vi "PH_Beamline.color ns-FE BL.vi"(0 "i ref in":refnum<vi>, 5 "error in (no error)":errorcluster) -> (14 "i ref out":refnum<vi>, 16 "Color State Exit ns-FE":i32, 19 "error out":errorcluster)   [LabVIEW 2014, in "PH_Beamline.lvlib"]
doc: "This VI colors the ns-Frontend beamline elements."
uses:
  PH_Beamline.lvlib
  PH_Basics/PH_SystemInformation/PH_SystemInformationEnabling State.ctl
  PH_Basics/PH_StatusHandler/PH_StatusHandler.Status.ctl
  PH_Basics/PH_Common/PH_Common.lvlib
  PH_Basics/PH_SystemInformation/PH_SystemInformation.lvlib
  PH_BL-Master/PH_BL-Master.lvlib
  PH_Basics/PH_StatusHandler/PH_StatusHandler.lvlib
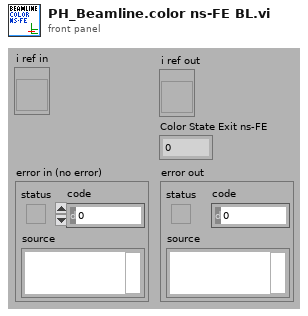
[diagram p1: front panel]
types:
  T1 = enum16{"Laser", "PreAmp", "MainAmp", "Exp 1", "Exp 2", "Exp 3", "Exp 4"}
  T2 = typedef "PH_StatusHandler.lvlib/PH_StatusHandler.Status.ctl" = i16
  T3 = typedef "PH_SystemInformation.lvlib/PH_SystemInformationEnabling State.ctl" = i32
  T4 = typedef "PH_Beamline.lvlib/PH_Beamline.i attribute.ctl" = cluster{"GUI Refs":cluster{"PA ok":refnum<vi>, "MA ok":refnum<vi>, "fs FE ok":refnum<vi>, "ns FE ok":refnum<vi>, "PA ED ok":refnum<vi>, "MAS ok":refnum<vi>, "Booster ok":refnum<vi>, "Mirrortower ok":refnum<vi>, "In.-Box ok":refnum<vi>, "Compressor ok":refnum<vi>, "Experiment LB ok":refnum<vi>, "Experiment LL ok":refnum<vi>, "PHELIX_Beckhoff_Watchdog":refnum<vi>, "Shutters closed":refnum<vi>, "uOPA ok":refnum<vi>, "Vacuum no shotcond Comp LB":refnum<vi>}, "Refs BL MA":refnum<vi>[], "Refs BL MA-IB":refnum<vi>[], "Refs BL fs":refnum<vi>[], "Refs BL PA ED":refnum<vi>[], "Refs BL MAS":refnum<vi>[], "Refs BL Boo":refnum<vi>[], "Refs BL ns":refnum<vi>[], "Refs BL Mirrortower":refnum<vi>[], "Refs BL Compressor":refnum<vi>[], "Refs BL Exp LB":refnum<vi>[], "Radiation Safety":cluster{"Exp Laserbay":cluster{"Ref Op Mode":refnum<vi>, "Ref Laserbay evacuated":refnum<vi>, "Tagname LB evacuated":string, "Shot Mode":T5, "Laserbay evacuated?":i32, "Tagname HV room locked":string, "HV room locked?":i32, "Ref HV room locked":refnum<vi>, "Tagname bridged?":string, "Ref Bridge":refnum<vi>, "I<1E18W/cm²":bool}, "Exp Laserlab":cluster{"Ref Op Mode":refnum<vi>, "Ref Laserlab evacuated":refnum<vi>, "Tagname LL evacuated":string, "Shot Mode":T5, "Laserlab evacuated?":i32, "Tagname bridged?":string, "Ref Bridge":refnum<vi>, "I<1E18W/cm²":bool}}, "Refs BL LL":refnum<vi>[], "PP Igni Heating GUI Refs":refnum<vi>[], "PP Igni Heating Tagnames ":string[], "Refs BL PA":cluster{"undelayed Line before Shutter":refnum<vi>[], "undelayed Line after Shutter":refnum<vi>[], "before Bypass":refnum<vi>[], "delayed Line before Shutter":refnum<vi>[], "delayed Line after Shutter":refnum<vi>[], "before Shutter Input":refnum<vi>[], "after Shutter Input":refnum<vi>[], "Bypass":refnum<vi>[], "before Shutter Exit":refnum<vi>[], "after Shutter Exit":refnum<vi>[], "to MA":refnum<vi>[], "to Lab":refnum<vi>[]}, "BL":cluster{"YLF_BL_Status":i32, "fs_BL_Status":i32, "fs_YLF_BL_Status":i32, "ns_BL_Status":i32, "PA_Input_BL_Status":i32, "PA_UnDelay_BL_Status":i32, "PA_Delay_BL_Status":i32, "PA_BL_Status":i32, "PA_Bypass_BL_Status":i32, "PA_Exit_BL_Status":i32, "PA_LL_BL_Status":i32, "LL_BL_Status":i32, "PA_MA_BL_Status":i32, "MA_Exit_BL_Status":i32, "MA_Z6_BL_Status":i32, "Z6_BL_Status":i32, "MA_LB_BL_Status":i32, "LB_TB2_BL_Status":i32, "PA_before_Bypass_BL_Status":i32, "LB_TB3_BL_Status":i32}, "State Subsystems":cluster{"PA":bool, "MA":bool, "ns FE":bool, "fs FE":bool, "PA ED":bool, "In.-Box":bool, "MAS":bool, "Booster":bool, "Mirrortower":bool, "Compressor":bool, "Experiment LB":bool, "Experiment LL":bool, "uOPA":bool}, "Status Subscriber Information":T6, "Refs BL uOPA":refnum<vi>[], "PA_Input_2_Beam_6PWpGUI not linked?":bool, "PA_Input_Delay_6PGUI not linked?":bool, "Settings":T9}
  T5 = typedef "PH_Beamline.lvlib/PH_Beamline.Operation Mode.ctl" = i32
  T6 = typedef "PH_Beamline.lvlib/PH_Beamline.Status Subscriber Information.ctl" = cluster{"fs Swich YLF":T7, "fs Exit Shutter":T7, "ns Exit Shutter":T7, "PA Input Shutter":T7, "PA PC WP":T7, "PA PC WP 2":T7, "PA Bypass In":T7, "PA Bypass Out":T7, "PA CH 1":T7, "PA delayed":T7, "PA non delayed":T7, "PA Exit Shutter":T7, "PA Switch Lab":T7, "PA Bridge CH Input MA":T7, "MA Diffusor IB":T7, "MA IB Ready":T7, "MA CH 1":T7, "MA CH 2":T7, "MA CH 3":T7, "MA CH 4":T7, "MA Shutter Align Cam":T7, "MA Position MM5":T7, "Calorimeter Switch":T7, "BL Z6 CH 9":T7, "BL Z6 Beamdump":T7, "BL Z6 Shutter":T7, "COS Sensitivity Switch":T7, "Exp LB Shutter":T7, "Exp LB TB 2":T7, "Exp LB TB 3":T7, "PA LL Input CH":T7, "PA LL Output CH":T7, "LL Comp Input Shutter":T7, "LL Comp Output Shutter":T7, "LL Comp FF Shutter":T7, "Exp LL Shutter":T7, "MA IM In IB":T7, "MA IM Out IB":T7, "MA DB In IB":T7, "MA DB Out IB":T7, "Exp LB Shutter Interlock":T7, "Exp LL Shutter Interlock":T7, "MM1 Force Sensor":T7}
  T7 = typedef "PH_BL-Master.lvlib/PH_BL-Master.Status Subscriber Information.ctl" = cluster{"Index of element":i32, "Attributeset":T8}
  T8 = typedef "PH_BL-Master.lvlib/PH_BL-Master.Attribute Set.ctl" = enum16{"Boolean Status Service Subscriber", "Picture Status Service Subscriber"}
  T9 = typedef "PH_Beamline_Chief.lvlib/PH_Beamline_Chief.Settings.ctl" = cluster{"PA Doublepass Mode":bool, "Compressor Vaccuum LB not relevant":bool, "Windowshutter TB2 not relevant":bool, "Windowshutter TB3 not relevant":bool}
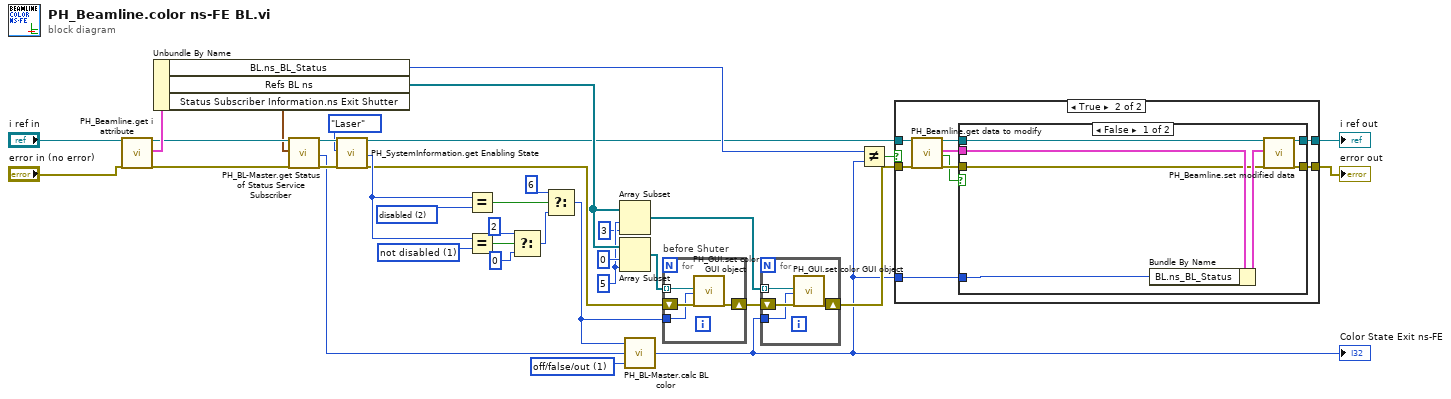
[diagram p0: block diagram]
diagram:
  w15 = T2 1 items=["no info", "off/false/out", "on/true/in", "Failure", "Alarm", "Status 1", "Status 2", "Status 3"] ("State for \"2\" (on) of ABLE (off/false/out)")
  w21 = T3 2 items=["no info", "not disabled", "disabled"] ("y")
  w22 = T3 1 items=["no info", "not disabled", "disabled"] ("y")
  w32 = 5 ("length")
  n1 = call "PH_Beamline.get i attribute.vi"("i ref in"="i ref in", "error in (no error)"="error in (no error)") -> ("i ref out"=w5:refnum<vi>, "i attribute"=w36:T4, "error out"=w4:errorcluster)  [unwired: 15 in]
  n2 = Unbundle By Name(w36) -> ("BL.ns_BL_Status"=w11:i32, "Refs BL ns"=w33:refnum<vi>[], "Status Subscriber Information.ns Exit Shutter"=w1:T7)
  n3 = call "PH_BL-Master.get Status of Status Service Subscriber.vi"("i ref in"=w5, "Wanted Status Subscriber Information"=w1, "error in (no error)"=w4) -> ("i ref out"=w27:refnum<vi>, "Status"=w16:T2, "error out"=w28:errorcluster)  [unwired: 11 in, 3 out]
  n4 = call "PH_SystemInformation.get Enabling State.vi"("i ref in"=w27, "Wanted State"=T1."Laser", "error in (no error)"=w28) -> ("i ref out"=w3:refnum<vi>, "Enabling State"=w24:T3, "error out"=w2:errorcluster)  [unwired: 14 in]
  n5 = Equal?(x=w24, y=w21) -> (x = y?=w26:bool)
  n6 = Equal?(x=w24, y=w22) -> (x = y?=w23:bool)
  n7 = Select(t=2 ("State before ABLE"), s=w23, f=0) -> (s? t:f=w19:i32)
  n8 = Select(t=6 ("State before ABLE"), s=w26, f=w19) -> (s? t:f=w17:i32)
  n9 = Array Subset(array=w33, index=w32, length=3) -> (w29:refnum<vi>[])
  n10 = Array Subset(array=w33, index=0, length=w32) -> (w34:refnum<vi>[])
  n11 = call "PH_BL-Master.calc BL color.vi"("State for \"2\" (on) of ABLE (off/false/out)"=w15, "State ABLE"=w16, "State before ABLE"=w17) -> ("State after ABLE"=w9:i32)
  "Color State Exit ns-FE" <- w9
  n12 = for "before Shuter" {
    tunnel: w34 -> [w40] mode=indexing
    shift-right: [w38] -> w30
    shift-left: w2 -> [w39]
    tunnel: w17 -> [w37]
    n13 = call "PH_GUI.set color GUI object.vi"("GUI object Ref"=w40, "State"=w37, "error in (no error)"=w39) -> ("error out"=w38:errorcluster)  [unwired: 16 in]
  }
  n14 = for {
    tunnel: w29 -> [w44] mode=indexing
    shift-right: [w42] -> w10
    shift-left: w30 -> [w43]
    tunnel: w9 -> [w41]
    n15 = call "PH_GUI.set color GUI object.vi"("GUI object Ref"=w44, "State"=w41, "error in (no error)"=w43) -> ("error out"=w42:errorcluster)  [unwired: 16 in]
  }
  n16 = Not Equal?(x=w11, y=w9) -> (x != y?=w14:bool)
  n17 = case shown="True" w14 {
    tunnel: w3 -> [w46 w51]
    tunnel: [w46 w50] -> w13
    tunnel: w10 -> [w45 w49]
    tunnel: [w45 w48] -> w12
    tunnel: w9 -> [_ w47]
    frame False {
    }
    frame True {
      n18 = call "PH_Beamline.get data to modify.vi"("i ref in"=w51, "error in (no error)"=w49) -> ("i ref out"=w54:refnum<vi>, "i attribute"=w52:T4, "timed out"=w53:bool, "error out"=w55:errorcluster)  [unwired: 14 in]
      n19 = case shown="False" w53 {
        tunnel: w55 -> [w56 w63]
        tunnel: w54 -> [w62 w64]
        tunnel: [w61 w63] -> w48
        tunnel: [w60 w64] -> w50
        tunnel: w52 -> [w57 _]
        tunnel: w47 -> [w58 _]
        frame False {
          n20 = Bundle By Name(cluster=w57, "BL.ns_BL_Status"=w58) -> (w59:T4)
          n21 = call "PH_Beamline.set modified data.vi"("i ref in"=w62, "i attribute"=w59, "error in (no error)"=w56) -> ("i ref out"=w60:refnum<vi>, "error out"=w61:errorcluster)  [unwired: 15 in]
        }
        frame True {
        }
      }
    }
  }
  "error out" <- w12
  "i ref out" <- w13
